vi "Marvin.vi"() -> ()   [LabVIEW 2017]
uses:
  Marvin ATP Remake 1.5.18/PCAN_Driver/ControlCAN.llb/CAN Channel.ctl
  Marvin ATP Remake 6.5.18 - Copy/PCAN_Driver/ControlCAN.llb/DevType.ctl
  Marvin ATP Remake 6.5.18/PCAN_Driver/ControlCAN.llb/VCI_INIT_CONFIG.ctl
  Marvin ATP Remake 6.5.18/PCAN_Driver/ControlCAN.llb/InitFlag.ctl
  Marvin ATP Remake 6.5.18/PCAN_Driver/ControlCAN.llb/Fliter.ctl
  Marvin ATP Remake 6.5.18/PCAN_Driver/ControlCAN.llb/Mode.ctl
  <vilib>/Utility/miscctls.llb/LVMinMaxIncTypeDef.ctl
  PCAN_Driver/ControlCAN.llb/VCI_CAN_OBJ.ctl
  PCAN_Driver/ControlCAN.lvlib
panel:
  in  "Clear Data Array":bool
  in  "PlayPause Data Array":bool
  out "CAN Data":cluster{"Frame Data":u64, "Frame ID":u32}[](array[cluster]) {"Frame ID" format="%.0x"; "Frame Data" format="%016x"}
  out "Waveform Chart":dbl[](graph)
  in  "Help Button":bool
  in  "Clear Monitor":bool
  out "Array":u64[][](array[numeric]) format="%016x"
  out "Ambient Over temp":bool
  out "Ambient Sensor temp":bool
  out "Ambient Temperature":dbl
  in  "Motor Over Temp":bool
  in  "Speed control":bool
  out "Unit Adress":string
  in  "Serial Send":bool
  in  "Index":u16(ring) items=["1"=1, "2"=2, "3"=3]
  out "read buffer":string
  in  "SetGet":enum16{"Get", "Set"}(ring)
  in  "Function":T1(ring)
  in  "Value":dbl
  in  "Value 1/2":enum16{"1", "2"}(ring)
  out "Msg Count":u32
  in  "Param to Set":u16(ring) items=["EBAY 5F"=95, "AHU 3F"=63, "AHU 2F"=47]
  out "UUT":u8
  out "Horizontal Progress Bar":i32(slide) min=0 max=48 scale=0.0..50.0
  in  "Set Param.":bool
  in  "Serial Monitor":bool caption="Graph Button"
  in  "Serial Com":bool
  in  "VISA resource name":refnum<visa-resource-name>="COM6"
  out "Serial Status":bool
  in  "Graph Button":bool
  in  "Refresh Button":bool
  out "Data Send":u64 format="%016x"
  in  "Motor Speed RPM":u16
  out "Under voltage/Over voltage":bool
  out "Speed error":bool
  out "Derated drive temp":bool
  out "Motor Over temperature":bool
  out "Commutation err":bool
  out "Motor Sensor temp Fauilre":bool
  out "Drive Over temperature":bool
  out "Drive Sensor temp Failure":bool
  out "Motor Phase Current RMS":dbl
  out "ECS State":u16
  out "Motor Speed RPM":dbl
  out "Motor Stator Temp.":dbl
  out "Power transistor Heat sink Temp.":dbl
  out "DC Current":dbl
  out "DC Voltage":dbl
  in  "Can Send":bool
  in  "Stop":bool
  out "Config_CANAT":T8 {"DevType" items=["USB-CAN"=3, "USB-CAN2"=4]; "CanIndex" items=["通道1", "通道2"]; "VCI_INIT_CONFIG"."Fliter" items=["接收所有类型"=3, "只接收标准帧"=4, "只接收扩展帧"=7]; "VCI_INIT_CONFIG"."Mode" items=["正常工作", "自测模式（环回）", "仅侦听模式"]; "VCI_INIT_CONFIG"."InitFlag" items=["使用Flash参数", "使用界面设置参数"]}
  in  "Channel 2":T3 caption="Channel" items=["Channel 1", "Channel 2"]
  out "CAN Status":bool
  out "Driver Version":string
  out "Hall Sensor Fault":bool
  out "Motor Phase Current":u16
  in  "Motor Phase Current":u16
  # "ver 1.7b"
  # "Marvin"
  # "REDLER TECHNOLOGIES LTD"
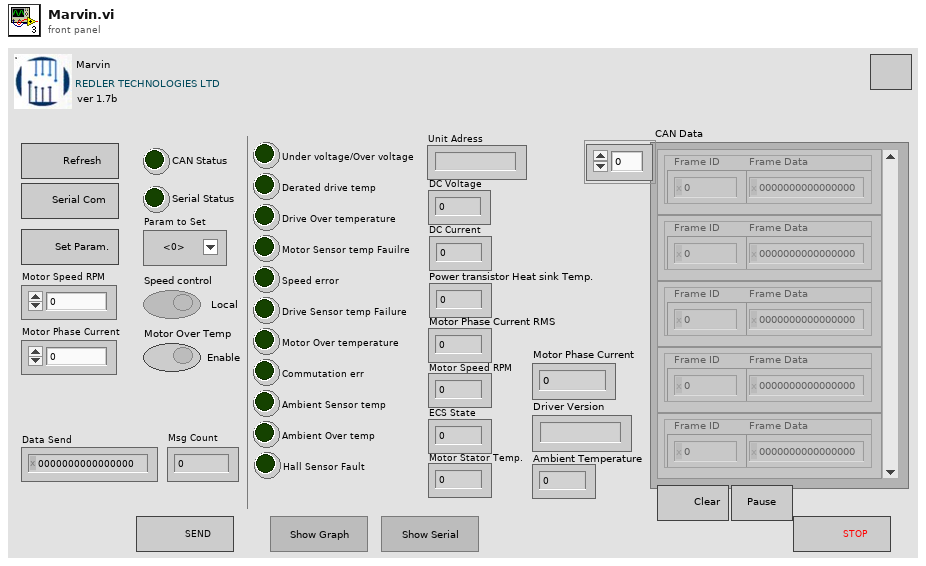
[diagram p1: front panel]
types:
  T1 = enum16{"Enable Conf. EP=1", "Serial Number", "Temperature", "Unit Adress", "Calibration", "Velocity", "Version"}
  T2 = typedef "ControlCAN.lvlib/DevType.ctl" = u32
  T3 = typedef "ControlCAN.lvlib/CAN Channel.ctl" = u32
  T4 = typedef "ControlCAN.lvlib/VCI_INIT_CONFIG.ctl" = cluster{"AccCode":u32, "AccMask":u32, "InitFlag":T5, "Fliter":T6, "Timing0":u8, "Timing1":u8, "Mode":T7}
  T5 = typedef "ControlCAN.lvlib/InitFlag.ctl" = u32
  T6 = typedef "ControlCAN.lvlib/Fliter.ctl" = u8
  T7 = typedef "ControlCAN.lvlib/Mode.ctl" = u8
  T8 = cluster{"DevType":T2, "DevIndex":u32, "CanIndex":T3, "VCI_INIT_CONFIG":T4}
  T9 = cluster{"ID":u32, "MSGTYPE":u8, "LEN":u8, "aDATA":u8[]}[]
  T10 = cluster{"ID":u32, "MSGTYPE":u8, "LEN":u8, "aDATA":u8[]}
  T11 = enum8{"Enabled", "Disabled", "Disabled and Grayed Out"}
  T12 = typedef "LVMinMaxIncTypeDef.ctl" = cluster{"Minimum":dbl, "Maximum":dbl, "Increment":dbl}
  T13 = enum32{"Invalid", "Standard", "Closed", "Hidden", "Minimized", "Maximized"}
  T14 = typedef "ControlCAN.lvlib/VCI_CAN_OBJ.ctl" = cluster{"ID":u32, "TimeStamp":u32, "TimeFlag":u8, "SendType":u8, "RemoteFlag":u8, "ExternFlag":u8, "DataLen":u8, "Data":u8[], "Reserved":u8[]}
  T15 = cluster{"Type":enum16{"接收", "发送"}, "Channel":T3, "Time":timestamp, "VCI_CAN_OBJ":T14}[]
  T16 = cluster{"Type":enum16{"接收", "发送"}, "Channel":T3, "Time":timestamp, "VCI_CAN_OBJ":T14}
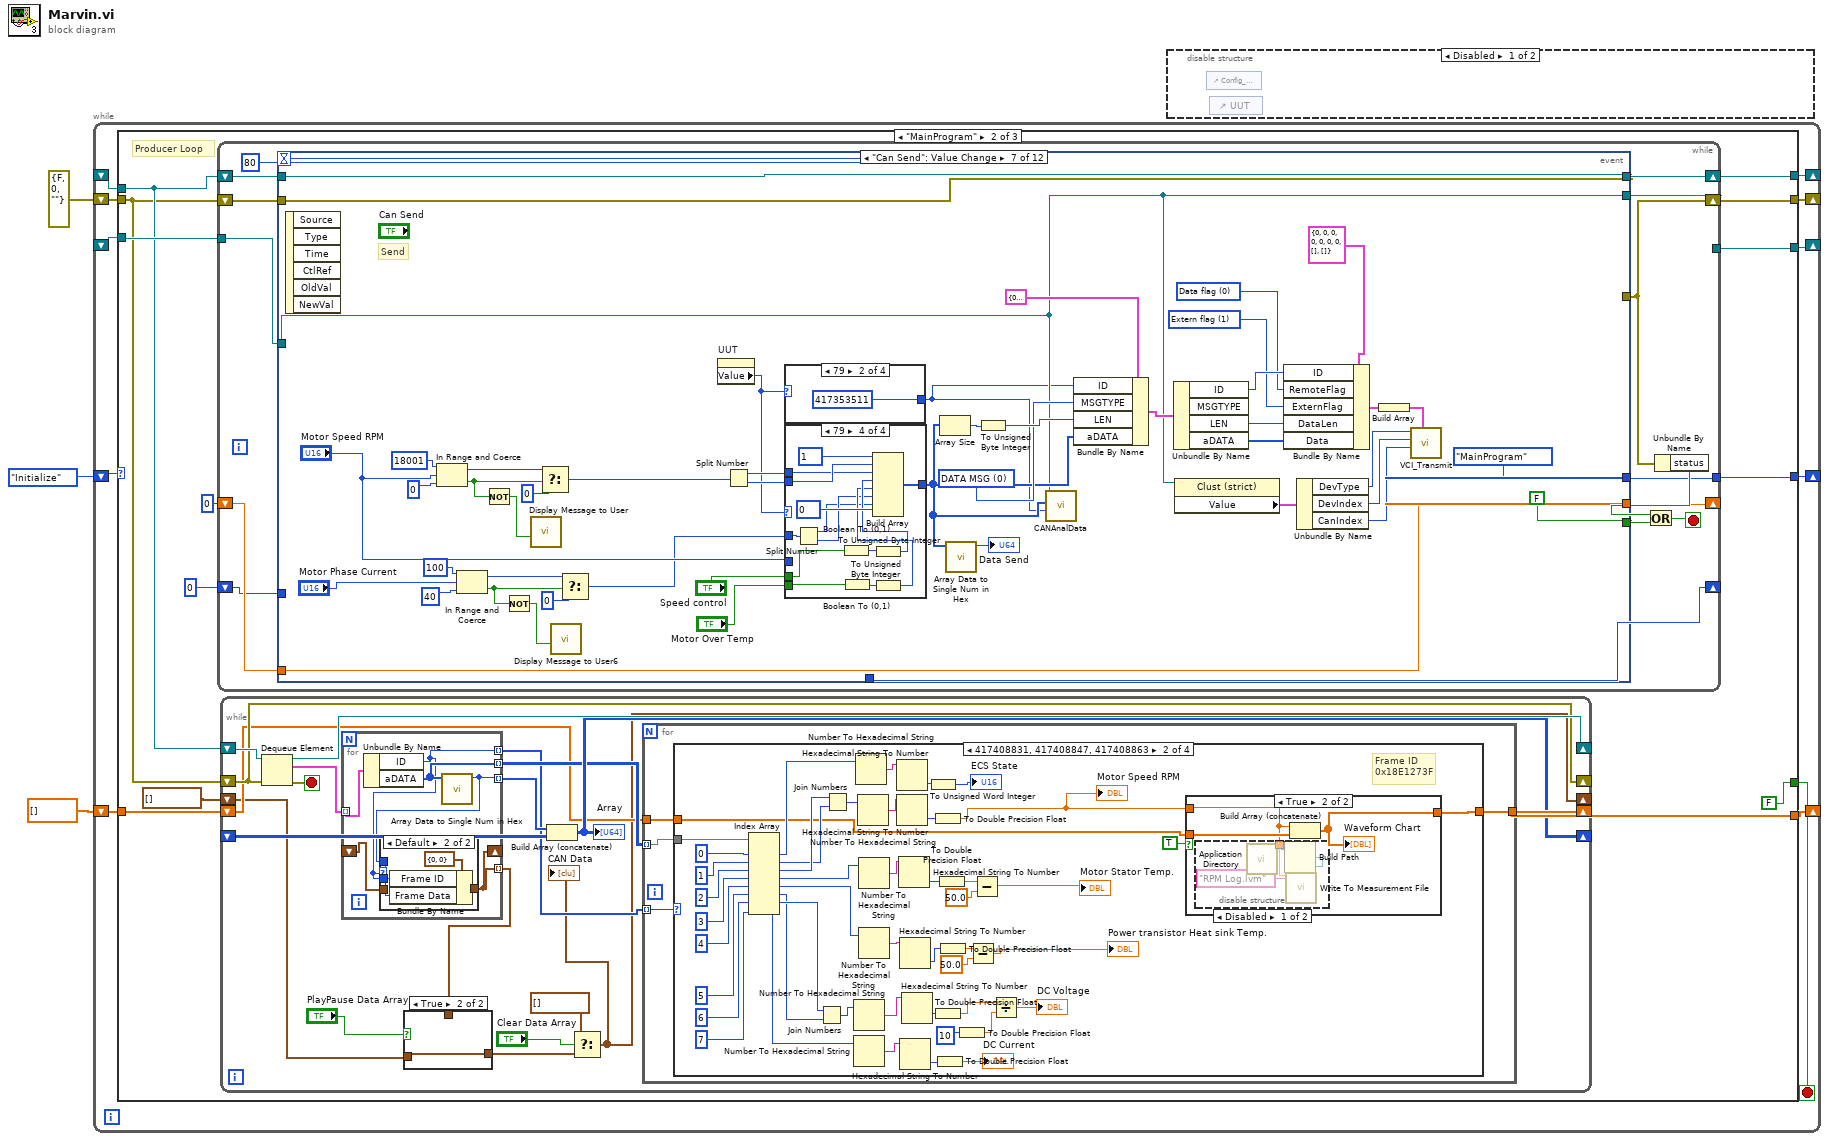
[diagram p0: block diagram]
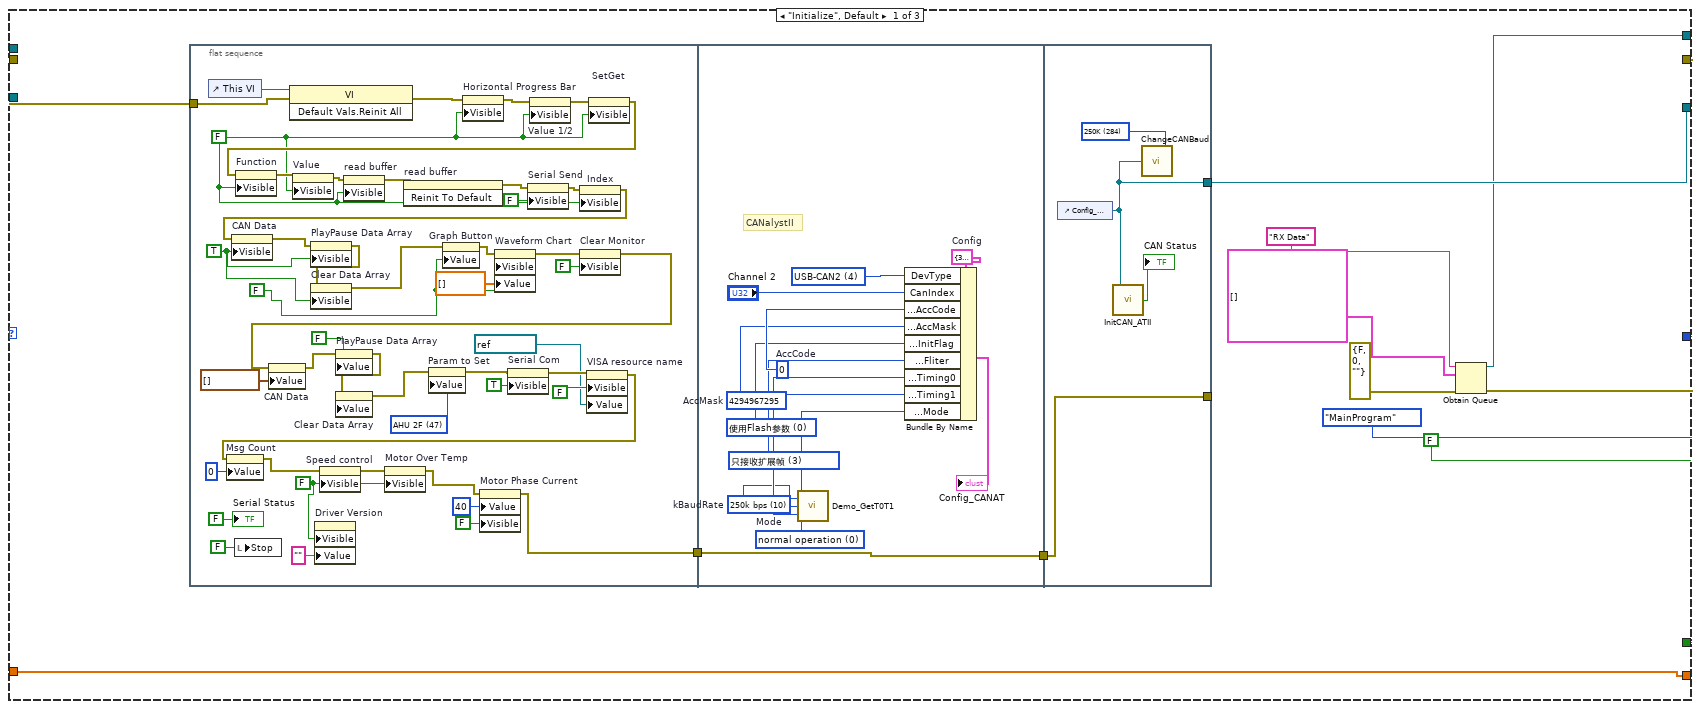
[diagram p3: hidden frame]
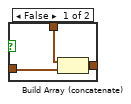
[diagram p4: hidden frame]
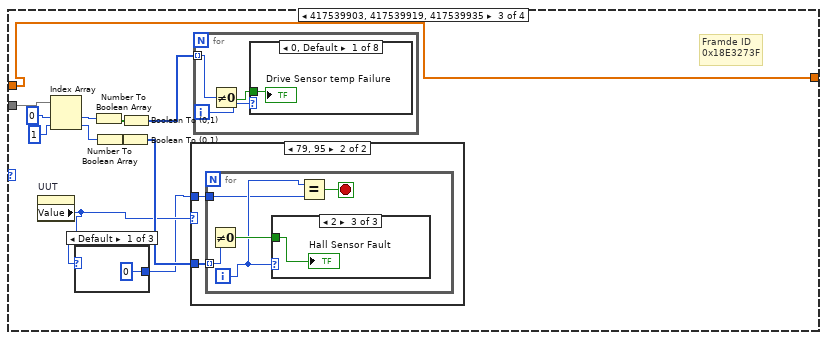
[diagram p8: hidden frame]
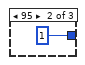
[diagram p9: hidden frame]
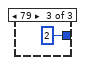
[diagram p10: hidden frame]
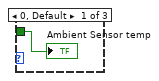
[diagram p12: hidden frame]
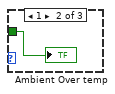
[diagram p13: hidden frame]
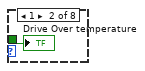
[diagram p14: hidden frame]
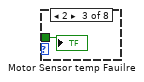
[diagram p15: hidden frame]
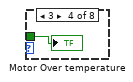
[diagram p16: hidden frame]
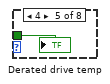
[diagram p17: hidden frame]
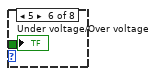
[diagram p18: hidden frame]
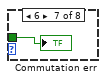
[diagram p19: hidden frame]
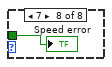
[diagram p20: hidden frame]
diagram:
  n1 = while {
    shift-right: [w9] -> _
    shift-left: enum16{"Stop", "MainProgram", "Initialize"}."Initialize" -> [w14]
    shift-right: [w13] -> _
    shift-left: _ -> [w12]
    shift-right: [w11] -> _
    shift-left: _ -> [w8]
    shift-right: [w10] -> _
    shift-left: errorcluster {"status"=FALSE, "code"=0, "source"=""} ("error out") -> [w7]
    shift-right: [w4] -> _
    shift-left: dbl[] [] -> [w5]
    stop <- w6 stop-if-true
    n2 = case shown="\"MainProgram\"" w14 {
      tunnel: [w26 w100 w995] -> w13
      tunnel: w12 -> [_ w103 w995]
      tunnel: [w22 w102 w996] -> w11
      tunnel: [w21 w101 w997] -> w10
      tunnel: [enum16{"Stop", "MainProgram", "Initialize"}."MainProgram" w99 enum16{"Stop", "MainProgram", "Initialize"}."Stop"] -> w9
      tunnel: w8 -> [_ w98 w996]
      tunnel: w7 -> [w19 w97 w998]
      tunnel: [FALSE ("Stop") FALSE ("Stop") w994] -> w6
      tunnel: w5 -> [w15 w94 w992]
      tunnel: [w15 w93 w992] -> w4
      frame "Initialize", Default {
        n3 = flat-sequence {
          tunnel: w19 -> [w55]
          tunnel: [w29] -> w17
          tunnel: [w74] -> w18
          tunnel: w17 -> [w74]
          tunnel: [w88] -> w26
          tunnel: w18 -> [w87]
          tunnel: [w87] -> _
          frame #0 {
            w38 = FALSE ("PlayPause Data Array")
            w32 = FALSE ("Visible")
            w65 = u16 47 items=["EBAY 5F"=95, "AHU 3F"=63, "AHU 2F"=47] ("Param to Set")
            w33 = TRUE ("Visible")
            w49 = FALSE ("Visible")
            w37 = FALSE ("Graph Button")
            n4 = control-ref of="This VI"() -> (w73:refnum<vi>)
            n5 = local write "Stop"(FALSE ("Stop")) -> ()
            n6 = invoke class="VI" method="Default Vals.Reinit All"(reference=w73, error in=w55) -> (error out=w54:errorcluster)  [unwired: 1 in, 2 out]
            n7 = property on="Driver Version" class="Str"("Visible"=w32, "Value"="" ("Driver Version")) -> ()  [unwired: 2 in, 2 out]
            n8 = property on="Horizontal Progress Bar" class="Slide (strict)"(error in=w54, "Visible"=w49) -> (error out=w63:errorcluster)  [unwired: 1 in, 1 out]
            n9 = property on="Value 1/2" class="Enum (strict)"(error in=w63, "Visible"=w49) -> (error out=w62:errorcluster)  [unwired: 1 in, 1 out]
            n10 = property on="SetGet" class="Enum (strict)"(error in=w62, "Visible"=w49) -> (error out=w61:errorcluster)  [unwired: 1 in, 1 out]
            n11 = property on="Function" class="Enum (strict)"(error in=w61, "Visible"=w49) -> (error out=w60:errorcluster)  [unwired: 1 in, 1 out]
            n12 = property on="Value" class="DigNum (strict)"(error in=w60, "Visible"=w49) -> (error out=w59:errorcluster)  [unwired: 1 in, 1 out]
            n13 = property on="read buffer" class="Str"(error in=w59, "Visible"=w49) -> (error out=w51:errorcluster)  [unwired: 1 in, 1 out]
            n14 = invoke on="read buffer" class="Str" method="Reinit To Default"(error in=w51) -> (error out=w50:errorcluster)  [unwired: 2 in, 2 out]
            n15 = property on="Serial Send" class="Bool (strict)"(error in=w50, "Visible"=FALSE) -> (error out=w58:errorcluster)  [unwired: 1 in, 1 out]
            n16 = property on="Index" class="Ring (strict)"(error in=w58, "Visible"=w49) -> (error out=w44:errorcluster)  [unwired: 1 in, 1 out]
            n17 = property on="CAN Data" class="Arr (strict)"(error in=w44, "Visible"=w33) -> (error out=w36:errorcluster)  [unwired: 1 in, 1 out]
            n18 = property on="PlayPause Data Array" class="Bool (strict)"(error in=w36, "Visible"=w33) -> (error out=w35:errorcluster)  [unwired: 1 in, 1 out]
            n19 = property on="Clear Data Array" class="Bool (strict)"(error in=w35, "Visible"=w33) -> (error out=w34:errorcluster)  [unwired: 1 in, 1 out]
            n20 = property on="Graph Button" class="Bool (strict)"(error in=w34, "Value"=w37) -> (error out=w47:errorcluster)  [unwired: 1 in, 1 out]
            n21 = property on="Waveform Chart" class="WFChart (strict)"(error in=w47, "Visible"=w37, "Value"=dbl[] [] ("Waveform Chart")) -> (error out=w46:errorcluster)  [unwired: 1 in, 1 out]
            n22 = property on="Clear Monitor" class="Bool"(error in=w46, "Visible"=FALSE) -> (error out=w43:errorcluster)  [unwired: 1 in, 1 out]
            n23 = property on="CAN Data" class="Arr (strict)"(error in=w43, "Value"=cluster{"Frame Data":u64, "Frame ID":u32}[] [] ("CAN Data")) -> (error out=w41:errorcluster)  [unwired: 1 in, 1 out]
            n24 = property on="PlayPause Data Array" class="Bool (strict)"(error in=w41, "Value"=w38) -> (error out=w40:errorcluster)  [unwired: 1 in, 1 out]
            n25 = property on="Clear Data Array" class="Bool (strict)"(error in=w40, "Value"=w38) -> (error out=w39:errorcluster)  [unwired: 1 in, 1 out]
            n26 = property on="Param to Set" class="Ring (strict)"(error in=w39, "Value"=w65) -> (error out=w57:errorcluster)  [unwired: 1 in, 1 out]
            n27 = property on="Serial Com" class="Bool"(error in=w57, "Visible"=TRUE) -> (error out=w70:errorcluster)  [unwired: 1 in, 1 out]
            n28 = property on="VISA resource name" class="VISAName"(error in=w70, "Visible"=FALSE, "Value"=refnum<visa-resource-name> "COM1" ("VISA resource name")) -> (error out=w56:errorcluster)  [unwired: 1 in, 1 out]
            n29 = property on="Msg Count" class="DigNum (strict)"(error in=w56, "Value"=u32 0 ("Msg Count")) -> (error out=w53:errorcluster)  [unwired: 1 in, 1 out]
            n30 = property on="Speed control" class="Bool (strict)"(error in=w53, "Visible"=w32) -> (error out=w52:errorcluster)  [unwired: 1 in, 1 out]
            n31 = property on="Motor Over Temp" class="Bool (strict)"(error in=w52, "Visible"=w32) -> (error out=w30:errorcluster)  [unwired: 1 in, 1 out]
            n32 = property on="Motor Phase Current" class="DigNum (strict)"(error in=w30, "Value"=u16 40 ("Motor Phase Current"), "Visible"=FALSE) -> (error out=w29:errorcluster)  [unwired: 1 in, 1 out]
            "Serial Status" <- FALSE ("Serial Status")
          }
          frame #1 {
            w78 = u32 4294967295  # AccMask
            w77 = T5 0 items=["使用Flash参数", "使用界面设置参数"] ("InitFlag")
            w75 = T7 0 items=["normal operation", "Listen-only mode", "test mode"]  # Mode
            w76 = T6 3 items=["接收所有类型"=1, "只接收标准帧"=2, "只接收扩展帧"=3] ("Fliter")
            w82 = u8 10 items=["5k bps"=1, "10k bps"=2, "20k bps"=3, "40k bps"=4, "50k bps"=5, "80k bps"=6, "100k bps"=7, "125k bps"=8, "200k bps"=9, "250k bps"=10, "400k bps"=11, "500k bps"=12, "666k bps"=13, "800k bps"=14, "1000k bps"=15, "33.33k bps"=16, "66.66k bps"=17, "83.33k bps"=18]  # kBaudRate
            w79 = u32 0  # AccCode
            w80 = T2 4 items=["USB-CAN"=3, "USB-CAN2"=4] ("DevType")
            w81 = T8 {"DevType"=3, "DevIndex"=0, "CanIndex"=0, "VCI_INIT_CONFIG"={"AccCode"=0, "AccMask"=0, "InitFlag"=1, "Fliter"=7, "Timing0"=0, "Timing1"=0, "Mode"=0}}  # Config
            # "CANalystII"
            n33 = call "Demo_GetT0T1.vi"("kBaudRate"=w82) -> ("Timing0"=w84:u8, "Timing1"=w85:u8)
            n34 = Bundle By Name(cluster=w81, "DevType"=w80, "CanIndex"="Channel 2", "VCI_INIT_CONFIG.AccCode"=w79, "VCI_INIT_CONFIG.AccMask"=w78, "VCI_INIT_CONFIG.InitFlag"=w77, "VCI_INIT_CONFIG.Fliter"=w76, "VCI_INIT_CONFIG.Timing0"=w84, "VCI_INIT_CONFIG.Timing1"=w85, "VCI_INIT_CONFIG.Mode"=w75) -> (→"Config_CANAT":T8)
          }
          frame #2 {
            w89 = u16 284 items=["1M"=20, "500K"=28, "250K"=284, "125K"=796, "100K"=17199, "50K"=18223, "20K"=21295, "10K"=26415, "5K"=32639] ("baud in")
            n35 = control-ref of="Config_CANAT"() -> (w88:refnum<vi>)
            n36 = call "InitCAN_ATII.vi"("Config"=w88) -> ("Sts"=→"CAN Status":bool)
            n37 = call "ChangeCANBaud.vi"("baud in"=w89, "reference"=w88) -> ()
          }
        }
        n38 = Obtain Queue(name (unnamed)="RX Data", element data type=T9 [], error in (no error)=errorcluster {"status"=FALSE, "code"=0, "source"=""}) -> (queue out=w22:refnum<queue>, error out=w21:errorcluster)  [unwired: 2 in, 1 out]
      }
      frame "MainProgram" {
        # "Producer Loop"
        n39 = while {
          shift-right: [w268] -> w101
          shift-left: w97 -> [w270]
          shift-right: [w269] -> w102
          shift-left: w98 -> [w271]
          tunnel: w103 -> [w272]
          tunnel: [w265] -> w100
          tunnel: [w264] -> w99
          shift-right: [w262] -> _
          shift-left: 0 -> [w263]
          shift-right: [w260] -> _
          shift-left: 0 -> [w261]
          stop <- w273 stop-if-true
          n40 = event shown="[6] \"Can Send\": Value Change" {
            selector: _ -> [_ _ _ _ _ _ _ _ _ _ _ _]
            dyn-events: _ -> [_ _ _ _ _ _ _ _ _ _ _ _]
            timeout: 80 ("Numeric") -> [_ _ _ _ _ _ _ _ _ _ _ _]
            tunnel: w272 -> [w294 w372 w391 w458 w713 w811 w841 w932 w952 w969 w984 w990]
            tunnel: w271 -> [w291 w373 w394 w459 w712 w812 w862 w933 w951 w970 w981 w987]
            tunnel: w270 -> [w276 w371 w389 w446 w705 w804 w861 w912 w947 w962 w980 w988]
            tunnel: [w289 w373 w394 w459 w712 w812 w862 w933 w951 w970 w979 w987] -> w269
            tunnel: [w288 w366 w390 w451 w701 w801 w861 w919 w944 w960 w977 w986] -> w268
            tunnel: [FALSE ("Stop") FALSE ("Stop") FALSE ("Stop") FALSE ("Stop") FALSE ("Stop") FALSE ("Stop") FALSE ("Stop") FALSE ("Stop") FALSE ("Stop") FALSE ("Stop") TRUE ("Stop") TRUE ("Stop")] -> w266
            tunnel: [w287 w372 w391 w458 w713 w811 w841 w932 w952 w969 w984 w990] -> w265
            tunnel: [enum16{"Stop", "MainProgram", "Initialize"}."MainProgram" enum16{"Stop", "MainProgram", "Initialize"}."MainProgram" enum16{"Stop", "MainProgram", "Initialize"}."MainProgram" enum16{"Stop", "MainProgram", "Initialize"}."MainProgram" enum16{"Stop", "MainProgram", "Initialize"}."MainProgram" enum16{"Stop", "MainProgram", "Initialize"}."MainProgram" enum16{"Stop", "MainProgram", "Initialize"}."MainProgram" enum16{"Stop", "MainProgram", "Initialize"}."MainProgram" enum16{"Stop", "MainProgram", "Initialize"}."MainProgram" enum16{"Stop", "MainProgram", "Initialize"}."MainProgram" enum16{"Stop", "MainProgram", "Initialize"}."Stop" enum16{"Stop", "MainProgram", "Initialize"}."Initialize"] -> w264
            tunnel: w263 -> [w283 w376 w387 w447 w703 w815 w827 w928 w943 w958 w976 w985]
            tunnel: [w282 w376 w387 w447 w703 w815 w827 w928 w943 w958 w976 w985] -> w262
            tunnel: w261 -> [w275 _ _ _ _ _ _ _ _ _ _ _]
            tunnel: [w275 _ _ _ _ _ _ _ _ _ _ _] -> w260
            event Timeout {
              n41 = event-data() -> ()  [unwired: 1 in, 3 out]
              n42 = property class="Clust (strict)"(reference=w294) -> (reference out=w287:refnum<vi>, "Value"=w295:T8)  [unwired: 1 in, 1 out]
              n43 = property on="Speed control" class="Bool (strict)"(error in=w276) -> ("Value"=w277:bool)  [unwired: 1 in, 2 out]
              n44 = case shown="True" w277 {
                frame False {
                }
                frame True {
                  n45 = property on="Motor Speed RPM" class="DigNum (strict)"() -> ("Value"=w301:u16)  [unwired: 2 in, 2 out]
                  n46 = control-ref of="Config_CANAT"() -> (w300:refnum<vi>)
                  n47 = control-ref of="UUT"() -> (w299:refnum<vi>)
                  n48 = call "CANSendMotorSpeed.vi"("Remote"=TRUE, "Motor Speed RPM"=w301, "UUT"=w299, "CAN Cluster in"=w300) -> ()  [unwired: 7 in, 1 out]
                }
              }
              n49 = Unbundle By Name(w295) -> ("DevType"=w296:T2, "CanIndex"=w292:T3)
              n50 = property on="Horizontal Progress Bar" class="Slide (strict)"(error in=w276, "Visible"=FALSE) -> (error out=w278:errorcluster)  [unwired: 1 in, 1 out]
              n51 = call "VCI_Receive.vi"("CANIndex"=w292, "DevIndex"=u32 0, "DevType"=w296) -> ("Recieve"=w290:T14[])  [unwired: 3 in, 5 out]
              n52 = Empty Array?(array=w290) -> (empty?=w293:bool)
              n53 = case shown="False" w293 {
                tunnel: w292 -> [w313 _]
                tunnel: w287 -> [w311 _]
                tunnel: w291 -> [w310 w365]
                tunnel: w278 -> [w309 w364]
                tunnel: w290 -> [w314 _]
                tunnel: [w304 w364] -> w288
                tunnel: [w303 w365] -> w289
                tunnel: [w302 0] -> w279
                frame False {
                  n54 = call "Demo_MakeDispBuff.vi"("Channel"=w313, "Type"=enum16{"接收", "发送"}."接收", "OBJs"=w314) -> ("Buffer"=w312:T15)
                  n55 = for {
                    N: 3 -> [_]
                    tunnel: w312 -> [w328]
                    tunnel: w311 -> [w327]
                    tunnel: w310 -> [w318]
                    tunnel: w309 -> [w317]
                    tunnel: [w320] -> w307 mode=indexing
                    tunnel: [w318] -> w306
                    tunnel: [w317] -> w305
                    tunnel: [w316] -> w302
                    i -> [w316]
                    n56 = property class="Clust (strict)"(reference=w327) -> ("Value"=w325:T8)  [unwired: 1 in, 2 out]
                    n57 = Index Array(array=w328, index=w316) -> (element=w321:T16)
                    n58 = Unbundle By Name(w321) -> ("Channel"=w323:T3, "VCI_CAN_OBJ"=w326:T14)  [unwired: 2 out]
                    n59 = Unbundle By Name(w325) -> ("CanIndex"=w324:T3)
                    n60 = Equal?(x=w324, y=w323) -> (x = y?=w322:bool)
                    n61 = case shown="True" w322 {
                      tunnel: w326 -> [_ w344]
                      tunnel: [w329 w340] -> w320
                      tunnel: T10 {"ID"=0, "MSGTYPE"=0, "LEN"=0, "aDATA"=[]} ("Msg") -> [w329 w339]
                      frame False {
                      }
                      frame True {
                        n62 = Unbundle By Name(w344) -> ("ID"=w338:u32, "DataLen"=w343:u8, "Data"=w341:u8[])
                        n63 = Bundle By Name(cluster=w339, "ID"=w338, "MSGTYPE"=u8 0, "LEN"=w343, "aDATA"=w341) -> (w340:T10)
                        n64 = Unbundle By Name(w340) -> ("ID"=w336:u32)
                        n65 = Split Number(x=w336) -> (lo(x)=w337:u16)  [unwired: 1 out]
                        n66 = Split Number(x=w337) -> (lo(x)=w334:u8)  [unwired: 1 out]
                        "UUT" <- w334
                        n67 = case shown="95" w334 {
                          tunnel: ["EBAY 5F" "PUMP 4F" w357 "AHU 3F" "AHU 2F"] -> w333
                          tunnel: [TRUE w354 w358 w359 w361] -> w331
                          tunnel: [TRUE w354 w356 w359 w361] -> w330
                          frame 95 {
                          }
                          frame 79 {
                            w354 = TRUE
                          }
                          frame Default {
                            n68 = property on="Hall Sensor Fault" class="Bool (strict)"() -> ("Visible"=w356:bool)  [unwired: 2 in, 2 out]
                            n69 = property on="Speed control" class="Bool (strict)"() -> ("Visible"=w358:bool)  [unwired: 2 in, 2 out]
                            n70 = property on="Unit Adress" class="Str"() -> ("Value"=w357:string)  [unwired: 2 in, 2 out]
                          }
                          frame 63 {
                            w359 = FALSE
                          }
                          frame 47 {
                            w361 = FALSE
                          }
                        }
                        n71 = Not Equal To 0?(x=w334) -> (x != 0?=w335:bool)
                        n72 = case shown="True" w335 {
                          tunnel: w334 -> [_ w350]
                          tunnel: w333 -> [_ w347]
                          tunnel: [w345 w346] -> w332
                          frame False {
                            n73 = property on="Unit Adress" class="Str"() -> ("Value"=w345:string)  [unwired: 2 in, 2 out]
                          }
                          frame True {
                            n74 = Number To Decimal String(number=w350) -> (decimal integer string=w349:string)  [unwired: 1 in]
                            n75 = call <vilib>:"Space Constant.vi"() -> ("String"=w348:string)
                            n76 = Concatenate Strings(w349, w348, w347) -> (w346:string)
                          }
                        }
                        "Unit Adress" <- w332
                        n77 = property on="Driver Version" class="Str"("Visible"=w331) -> ()  [unwired: 2 in, 2 out]
                        n78 = property on="Hall Sensor Fault" class="Bool (strict)"("Visible"=w330) -> ()  [unwired: 2 in, 2 out]
                        n79 = property on="Motor Phase Current" class="DigNum (strict)"("Visible"=w330) -> ()  [unwired: 2 in, 2 out]
                        n80 = property on="Motor Phase Current" class="DigNum (strict)"("Visible"=w330) -> ()  [unwired: 2 in, 2 out]
                        n81 = property on="Ambient Over temp" class="Bool (strict)"("Visible"=w331) -> ()  [unwired: 2 in, 2 out]
                        n82 = property on="Ambient Sensor temp" class="Bool (strict)"("Visible"=w331) -> ()  [unwired: 2 in, 2 out]
                        n83 = property on="Ambient Temperature" class="DigNum (strict)"("Visible"=w331) -> ()  [unwired: 2 in, 2 out]
                        n84 = property on="Motor Over Temp" class="Bool (strict)"("Visible"=w331) -> ()  [unwired: 2 in, 2 out]
                        n85 = property on="Speed control" class="Bool (strict)"("Visible"=w331) -> ()  [unwired: 2 in, 2 out]
                      }
                    }
                  }
                  n86 = Enqueue Element(queue=w306, element=w307, error in (no error)=w305) -> (queue out=w303:refnum<queue>, error out=w304:errorcluster)  [unwired: 2 out]
                }
                frame True {
                }
              }
              n87 = Divide(x=w279, y=u32 2) -> (x/y=w280:dbl)
              n88 = Add(x=w280, y=w283) -> (x+y=w282:dbl)
              "Msg Count" <- w282
            }
            event "Clear Monitor": Value Change {
              n89 = event-data() -> ()  [unwired: 1 in, 6 out]
              n90 = property on="VISA resource name" class="VISAName"(error in=w371) -> (error out=w370:errorcluster, "Value"=w369:refnum<visa-resource-name>)  [unwired: 1 in, 1 out]
              n91 = disable-structure shown="Enabled" {
                disable-tunnel: w370 -> [w381 w384]
                disable-tunnel: w369 -> [w379 w385]
                disable-tunnel: [w378 ""] -> w368
                disable-tunnel: [w377 w383] -> w367
                frame Disabled {
                  n92 = call "Serial.vi"("error in (no error)"=w381, "Clear Log"=TRUE, "VISA resource name"=w379) -> ("error out"=w377:errorcluster, "read buffer"=w378:string)  [unwired: 7 in]
                }
                frame Enabled {
                  n93 = VISA Flush I/O Buffer(VISA resource name=w385, error in (no error)=w384) -> (error out=w383:errorcluster)  [unwired: 1 in, 1 out]
                }
              }
              n94 = property on="read buffer" class="Str"(error in=w367, "Value"=w368) -> (error out=w366:errorcluster)  [unwired: 1 in, 1 out]
            }
            event "Serial Monitor": Value Change {
              n95 = event-data() -> ()  [unwired: 1 in, 6 out]
              n96 = property on="Serial Status" class="Bool (strict)"(error in=w389) -> (error out=w388:errorcluster, "Value"=w386:bool)  [unwired: 1 in, 1 out]
              n97 = case shown="True" w386 {
                tunnel: w388 -> [w398 w411]
                tunnel: [w396 w416] -> w390
                frame False {
                  n98 = call "Display Message to User3"("error in (no error)"=w398) -> ("error out"=w397:errorcluster)  [unwired: 9 in, 1 out]
                  n99 = property on="Serial Monitor" class="Bool (strict)"(error in=w397, "Value"=FALSE ("Serial Monitor")) -> (error out=w396:errorcluster)  [unwired: 1 in, 1 out]
                }
                frame True {
                  w403 = FALSE ("Visible")
                  w413 = FALSE ("Visible")
                  w414 = u16 1 items=["1"=1, "2"=2, "3"=3] ("Index")
                  n100 = property on="Index" class="Ring (strict)"(error in=w411, "Value"=w414) -> (error out=w410:errorcluster)  [unwired: 1 in, 1 out]
                  n101 = property on="Value 1/2" class="Enum (strict)"(error in=w410, "Visible"=w413) -> (error out=w409:errorcluster)  [unwired: 1 in, 1 out]
                  n102 = property on="Value" class="DigNum (strict)"(error in=w409, "Visible"=w413) -> (error out=w408:errorcluster)  [unwired: 1 in, 1 out]
                  n103 = property on="SetGet" class="Enum (strict)"(error in=w408, "Value"=enum16{"Get", "Set"}."Get" ("SetGet")) -> (error out=w407:errorcluster)  [unwired: 1 in, 1 out]
                  n104 = property on="Serial Send" class="Bool (strict)"(error in=w407, "Visible"=w403) -> (error out=w402:errorcluster)  [unwired: 1 in, 1 out]
                  n105 = property on="Clear Monitor" class="Bool"(error in=w402, "Visible"=w403) -> (error out=w401:errorcluster)  [unwired: 1 in, 1 out]
                  n106 = property on="Function" class="Enum (strict)"(error in=w401, "Value"=T1."Serial Number" ("Function")) -> (error out=w406:errorcluster)  [unwired: 1 in, 1 out]
                  n107 = property on="Index" class="Ring (strict)"(error in=w406, "DisabledEnum"=T11."Disabled and Grayed Out" ("Disabled")) -> (error out=w404:errorcluster)  [unwired: 1 in, 1 out]
                  n108 = case shown="True" "Serial Monitor" {
                    selector: "Serial Monitor" -> [w420 w441]
                    tunnel: w404 -> [w419 w437]
                    tunnel: [w422 w438] -> w416
                    tunnel: [FALSE TRUE] -> w400
                    frame False {
                      n109 = property on="Graph Button" class="Bool (strict)"(error in=w419) -> (error out=w418:errorcluster, "Value"=w417:bool)  [unwired: 1 in, 1 out]
                      n110 = case shown="True" w417 {
                        tunnel: [w426 w431] -> w423
                        tunnel: w418 -> [w428 w434]
                        tunnel: w420 -> [w429 _]
                        frame False {
                          n111 = property on="Waveform Chart" class="WFChart (strict)"(error in=w428, "Visible"=FALSE) -> (error out=w425:errorcluster)  [unwired: 1 in, 1 out]
                          n112 = Not(x=w429) -> (.not. x?=w424:bool)
                          n113 = property on="PlayPause Data Array" class="Bool (strict)"("Visible"=w424) -> ()  [unwired: 2 in, 2 out]
                          n114 = property on="Clear Data Array" class="Bool (strict)"("Visible"=w424) -> ()  [unwired: 2 in, 2 out]
                          n115 = property on="CAN Data" class="Arr (strict)"(error in=w425, "Visible"=w424) -> (error out=w426:errorcluster)  [unwired: 1 in, 1 out]
                        }
                        frame True {
                          w430 = FALSE ("Visible")
                          n116 = property on="Waveform Chart" class="WFChart (strict)"(error in=w434, "Visible"=TRUE) -> (error out=w432:errorcluster)  [unwired: 1 in, 1 out]
                          n117 = property on="PlayPause Data Array" class="Bool (strict)"("Visible"=w430) -> ()  [unwired: 2 in, 2 out]
                          n118 = property on="Clear Data Array" class="Bool (strict)"("Visible"=w430) -> ()  [unwired: 2 in, 2 out]
                          n119 = property on="CAN Data" class="Arr (strict)"(error in=w432, "Visible"=w430) -> (error out=w431:errorcluster)  [unwired: 1 in, 1 out]
                        }
                      }
                      n120 = property on="Serial Monitor" class="Bool (strict)"(error in=w423, "Value"=w420) -> (error out=w422:errorcluster)  [unwired: 1 in, 1 out]
                    }
                    frame True {
                      n121 = Not(x=w441) -> (.not. x?=w435:bool)
                      n122 = property on="PlayPause Data Array" class="Bool (strict)"("Visible"=w435) -> ()  [unwired: 2 in, 2 out]
                      n123 = property on="CAN Data" class="Arr (strict)"(error in=w437, "Visible"=w435) -> (error out=w436:errorcluster)  [unwired: 1 in, 1 out]
                      n124 = property on="Clear Data Array" class="Bool (strict)"("Visible"=w435) -> ()  [unwired: 2 in, 2 out]
                      n125 = property on="Serial Monitor" class="Bool (strict)"(error in=w436, "Value"=w441) -> (error out=w440:errorcluster)  [unwired: 1 in, 1 out]
                      n126 = property on="Graph Button" class="Bool (strict)"(error in=w440, "Value"=w435) -> (error out=w439:errorcluster)  [unwired: 1 in, 1 out]
                      n127 = property on="Waveform Chart" class="WFChart (strict)"(error in=w439, "Visible"=w435) -> (error out=w438:errorcluster)  [unwired: 1 in, 1 out]
                    }
                  }
                  n128 = property on="SetGet" class="Enum (strict)"("Visible"=w400) -> ()  [unwired: 2 in, 2 out]
                  n129 = property on="Index" class="Ring (strict)"("Visible"=w400) -> ()  [unwired: 2 in, 2 out]
                  n130 = property on="Function" class="Enum (strict)"("Visible"=w400) -> ()  [unwired: 2 in, 2 out]
                  n131 = property on="Clear Monitor" class="Bool"("Visible"=w400) -> ()  [unwired: 2 in, 2 out]
                  n132 = property on="Serial Send" class="Bool (strict)"("Visible"=w400) -> ()  [unwired: 2 in, 2 out]
                  n133 = property on="read buffer" class="Str"("Visible"=w400) -> ()  [unwired: 2 in, 2 out]
                }
              }
            }
            event "Serial Send", "Function", "SetGet": Value Change {
              n134 = event-data() -> ()  [unwired: 1 in, 6 out]
              n135 = case shown="\"Enable Conf. EP=1\"" "Function" {
                tunnel: w446 -> [w465 w470 w477 w479 w482 w486 w488 w489]
                tunnel: [w464 w472 w476 w481 w484 w485 w488 w489] -> w444
                frame "Serial Number" {
                  n136 = property on="Index" class="Ring (strict)"(error in=w465, "DisabledEnum"=T11."Disabled and Grayed Out" ("Disabled")) -> (error out=w464:errorcluster)  [unwired: 1 in, 1 out]
                }
                frame "Temperature" {
                  n137 = property on="UUT" class="DigNum (strict)"() -> ("Value"=w467:u8)  [unwired: 2 in, 2 out]
                  n138 = case shown="95" w467 {
                    tunnel: [i32[] [2] ("Disabled Items []") i32[] [3] ("Disabled Items []")] -> w468
                    frame 47, 63, Default {
                    }
                    frame 95 {
                    }
                  }
                  n139 = property on="Index" class="Ring (strict)"(error in=w470, "DisabledEnum"=T11."Enabled" ("Disabled"), "Visible"=TRUE, "Disabled Items []"=w468) -> (error out=w472:errorcluster)  [unwired: 1 in, 1 out]
                }
                frame "Unit Adress" {
                  n140 = property on="Index" class="Ring (strict)"(error in=w477, "DisabledEnum"=T11."Enabled" ("Disabled"), "Visible"=TRUE) -> (error out=w476:errorcluster)  [unwired: 1 in, 1 out]
                }
                frame "Calibration" {
                  n141 = property on="Index" class="Ring (strict)"(error in=w479, "DisabledEnum"=T11."Disabled and Grayed Out" ("Disabled")) -> (error out=w481:errorcluster)  [unwired: 1 in, 1 out]
                }
                frame "Velocity" {
                  n142 = property on="Index" class="Ring (strict)"(error in=w482, "DisabledEnum"=T11."Disabled and Grayed Out" ("Disabled")) -> (error out=w484:errorcluster)  [unwired: 1 in, 1 out]
                }
                frame "Version" {
                  n143 = property on="Index" class="Ring (strict)"(error in=w486, "DisabledEnum"=T11."Disabled and Grayed Out" ("Disabled")) -> (error out=w485:errorcluster)  [unwired: 1 in, 1 out]
                }
                frame "Enable Conf. EP=1" {
                }
                frame Default {
                }
              }
              n144 = property on="VISA resource name" class="VISAName"() -> ("Value"=w460:refnum<visa-resource-name>)  [unwired: 2 in, 2 out]
              n145 = property on="read buffer" class="Str"(error in=w444) -> (error out=w453:errorcluster, "Text.Scroll Position"=w450:u32)  [unwired: 1 in, 1 out]
              n146 = case shown="\"Set\"" "SetGet" {
                tunnel: "Function" -> [w493 w592]
                tunnel: w460 -> [w499 w602]
                tunnel: w453 -> [w496 w591]
                tunnel: "Value" -> [_ w601]
                tunnel: "Value 1/2" -> [_ w599]
                tunnel: "Index" -> [w494 w596]
                tunnel: [w498 w594] -> w452
                tunnel: [w491 w593] -> w457
                tunnel: "Serial Send" -> [w490 w583]
                frame "Get", Default {
                  w497 = FALSE ("Visible")
                  n147 = property on="Value" class="DigNum (strict)"(error in=w496, "Visible"=w497) -> (error out=w495:errorcluster)  [unwired: 1 in, 1 out]
                  n148 = property on="Value 1/2" class="Enum (strict)"(error in=w495, "Visible"=w497) -> (error out=w492:errorcluster)  [unwired: 1 in, 1 out]
                  n149 = case shown="True" w490 {
                    tunnel: w499 -> [_ w510]
                    tunnel: [w500 w505] -> w498
                    tunnel: w494 -> [_ w509]
                    tunnel: w493 -> [_ w508]
                    tunnel: w492 -> [w500 w507]
                    tunnel: [w501 w503] -> w491
                    frame False {
                      n150 = property on="read buffer" class="Str"() -> ("Value"=w501:string)  [unwired: 2 in, 2 out]
                    }
                    frame True {
                      n151 = case shown="\"Serial Number\"" w508 {
                        tunnel: w510 -> [w515 w533 w549 w558 w565 w576 _]
                        tunnel: w507 -> [w513 w524 w539 w553 w563 w574 w581]
                        tunnel: [w518 w534 w550 w559 w569 w577 w581] -> w505
                        tunnel: [w517 w535 w548 w560 w570 w572 "Cannot perform operation.\n" ("read buffer")] -> w504
                        tunnel: w509 -> [_ w528 w541 _ _ _ _]
                        frame "Serial Number" {
                          n152 = property on="Index" class="Ring (strict)"(error in=w513, "DisabledEnum"=T11."Disabled and Grayed Out" ("Disabled")) -> (error out=w512:errorcluster)  [unwired: 1 in, 1 out]
                          n153 = Concatenate Strings("SN" ("string"), "\r\n" ("write buffer")) -> (w516:string)
                          n154 = call "Serial.vi"("error in (no error)"=w512, "Clear Log"=FALSE, "write buffer"=w516, "VISA resource name"=w515) -> ("error out"=w518:errorcluster, "read buffer"=w517:string)  [unwired: 6 in]
                        }
                        frame "Temperature" {
                          n155 = Number To Decimal String(number=w528) -> (decimal integer string=w527:string)  [unwired: 1 in]
                          n156 = property on="Index" class="Ring (strict)"(error in=w524, "DisabledEnum"=T11."Enabled" ("Disabled"), "Visible"=TRUE) -> (error out=w523:errorcluster)  [unwired: 1 in, 1 out]
                          n157 = Concatenate Strings("TA" ("string"), "[", w527, "]", "\r\n" ("write buffer")) -> (w529:string)
                          n158 = call "Serial.vi"("error in (no error)"=w523, "Clear Log"=FALSE, "write buffer"=w529, "VISA resource name"=w533) -> ("error out"=w534:errorcluster, "read buffer"=w535:string)  [unwired: 6 in]
                        }
                        frame "Unit Adress" {
                          n159 = Number To Decimal String(number=w541) -> (decimal integer string=w547:string)  [unwired: 1 in]
                          n160 = property on="Index" class="Ring (strict)"(error in=w539, "DisabledEnum"=T11."Enabled" ("Disabled"), "Visible"=TRUE) -> (error out=w538:errorcluster)  [unwired: 1 in, 1 out]
                          n161 = Concatenate Strings("UA" ("string"), "[", w547, "]", "\r\n" ("write buffer")) -> (w542:string)
                          n162 = call "Serial.vi"("error in (no error)"=w538, "Clear Log"=FALSE, "write buffer"=w542, "VISA resource name"=w549) -> ("error out"=w550:errorcluster, "read buffer"=w548:string)  [unwired: 6 in]
                        }
                        frame "Calibration" {
                          n163 = property on="Index" class="Ring (strict)"(error in=w553, "DisabledEnum"=T11."Disabled and Grayed Out" ("Disabled")) -> (error out=w552:errorcluster)  [unwired: 1 in, 1 out]
                          n164 = Concatenate Strings("CC" ("string"), "\r\n" ("write buffer")) -> (w556:string)
                          n165 = call "Serial.vi"("error in (no error)"=w552, "Clear Log"=FALSE, "write buffer"=w556, "VISA resource name"=w558) -> ("error out"=w559:errorcluster, "read buffer"=w560:string)  [unwired: 6 in]
                        }
                        frame "Velocity" {
                          n166 = property on="Index" class="Ring (strict)"(error in=w563, "DisabledEnum"=T11."Disabled and Grayed Out" ("Disabled")) -> (error out=w562:errorcluster)  [unwired: 1 in, 1 out]
                          n167 = Concatenate Strings("VC" ("string"), "\r\n" ("write buffer")) -> (w566:string)
                          n168 = call "Serial.vi"("error in (no error)"=w562, "Clear Log"=FALSE, "write buffer"=w566, "VISA resource name"=w565) -> ("error out"=w569:errorcluster, "read buffer"=w570:string)  [unwired: 6 in]
                        }
                        frame "Version" {
                          n169 = Concatenate Strings("VR" ("string"), "\r\n" ("write buffer")) -> (w578:string)
                          n170 = property on="Index" class="Ring (strict)"(error in=w574, "DisabledEnum"=T11."Disabled and Grayed Out" ("Disabled")) -> (error out=w573:errorcluster)  [unwired: 1 in, 1 out]
                          n171 = call "Serial.vi"("error in (no error)"=w573, "Clear Log"=FALSE, "write buffer"=w578, "VISA resource name"=w576) -> ("error out"=w577:errorcluster, "read buffer"=w572:string)  [unwired: 6 in]
                        }
                        frame Default {
                        }
                      }
                      n172 = property on="Serial Send" class="Bool (strict)"(error in=w505, "Value"=FALSE ("Serial Send")) -> ()  [unwired: 1 in, 2 out]
                      n173 = property on="read buffer" class="Str"() -> ("Value"=w502:string)  [unwired: 2 in, 2 out]
                      n174 = Concatenate Strings(w502, w504) -> (w503:string)
                    }
                  }
                }
                frame "Set" {
                  n175 = To Unsigned Long Integer(number=w601) -> (unsigned 32bit integer=w597:u32)
                  n176 = Number To Decimal String(number=w596) -> (decimal integer string=w595:string)  [unwired: 1 in]
                  n177 = Number To Decimal String(number=w599) -> (decimal integer string=w598:string)  [unwired: 1 in]
                  n178 = case shown="Default" w592 {
                    tunnel: w591 -> [w676 w680 w684 w688 w692 w696 w698 w700]
                    tunnel: [FALSE TRUE TRUE FALSE FALSE FALSE w697 w699] -> w589
                    tunnel: [TRUE TRUE TRUE FALSE TRUE FALSE w697 w699] -> w588
                    tunnel: [FALSE FALSE FALSE TRUE FALSE FALSE w697 w699] -> w587
                    tunnel: [w676 w680 w684 w688 w692 w696 w698 w700] -> w585
                    frame "Serial Number" {
                    }
                    frame "Temperature" {
                    }
                    frame "Unit Adress" {
                    }
                    frame "Calibration" {
                    }
                    frame "Velocity" {
                    }
                    frame "Version" {
                    }
                    frame "Enable Conf. EP=1" {
                      w697 = FALSE
                    }
                    frame Default {
                      w699 = FALSE
                    }
                  }
                  n179 = Number To Decimal String(number=w597) -> (decimal integer string=w600:string)  [unwired: 1 in]
                  n180 = property on="Index" class="Ring (strict)"(error in=w585, "Visible"=w589) -> (error out=w590:errorcluster)  [unwired: 1 in, 1 out]
                  n181 = property on="Value" class="DigNum (strict)"(error in=w590, "Visible"=w588) -> (error out=w586:errorcluster)  [unwired: 1 in, 1 out]
                  n182 = property on="Value 1/2" class="Enum (strict)"(error in=w586, "Visible"=w587) -> (error out=w584:errorcluster)  [unwired: 1 in, 1 out]
                  n183 = case shown="True" w583 {
                    tunnel: w602 -> [_ w616]
                    tunnel: w600 -> [_ w615]
                    tunnel: w598 -> [_ w614]
                    tunnel: w597 -> [_ w613]
                    tunnel: w595 -> [_ w612]
                    tunnel: [w603 w611] -> w594
                    tunnel: [w604 w610] -> w593
                    tunnel: w592 -> [_ w608]
                    tunnel: w584 -> [w603 w607]
                    frame False {
                      n184 = property on="read buffer" class="Str"() -> ("Value"=w604:string)  [unwired: 2 in, 2 out]
                    }
                    frame True {
                      n185 = flat-sequence {
                        tunnel: [w620] -> w618
                        tunnel: w607 -> [w620]
                        frame #0 {
                          n186 = Wait (ms)(milliseconds to wait=u32 50) -> ()  [unwired: 1 out]
                        }
                      }
                      n187 = case shown="\"Velocity\"" w608 {
                        tunnel: [w623 w629 w638 w646 w664 "EP=1\r\n" ("write buffer") "Cannot perform operation.\n" ("read buffer")] -> w609
                        tunnel: w618 -> [w622 w628 w637 w651 w655 w667 w669]
                        tunnel: [w622 w628 w637 w651 w652 w667 w669] -> w617
                        tunnel: w615 -> [w624 w630 w643 _ _ _ _]
                        tunnel: w614 -> [_ _ _ w647 _ _ _]
                        tunnel: w613 -> [_ _ _ _ w656 _ _]
                        tunnel: w612 -> [_ w631 w641 _ _ _ _]
                        frame "Serial Number" {
                          n188 = Concatenate Strings("SN" ("write buffer"), "=" ("string"), w624, "\r\n" ("write buffer")) -> (w623:string)
                        }
                        frame "Temperature" {
                          n189 = Concatenate Strings("TA" ("string"), "[", w631, "]", "=" ("string"), w630, "\r\n" ("write buffer")) -> (w629:string)
                        }
                        frame "Unit Adress" {
                          n190 = Concatenate Strings("UA" ("string"), "[", w641, "]", "=" ("string"), w643, "\r\n" ("write buffer")) -> (w638:string)
                        }
                        frame "Calibration" {
                          n191 = Concatenate Strings("CC" ("string"), "=" ("string"), w647, "\r\n" ("write buffer")) -> (w646:string)
                        }
                        frame "Velocity" {
                          n192 = In Range and Coerce(upper limit=u16 18001, x=w656, lower limit=u16 0) -> (coerced(x)=w662:u32, In Range?=w660:bool)
                          n193 = Not(x=w660) -> (.not. x?=w661:bool)
                          n194 = Select(t=w662, s=w660, f=u16 0) -> (s? t:f=w654:u32)
                          n195 = Number To Decimal String(number=w654) -> (decimal integer string=w653:string)  [unwired: 1 in]
                          n196 = Concatenate Strings("VC" ("write buffer"), "=" ("string"), w653, "\r\n" ("write buffer")) -> (w664:string)
                          n197 = call "Display Message to User2"("error in (no error)"=w655, "Enable"=w661) -> ("error out"=w652:errorcluster)  [unwired: 8 in, 1 out]
                        }
                        frame "Enable Conf. EP=1" {
                        }
                        frame Default {
                        }
                      }
                      n198 = property on="read buffer" class="Str"() -> ("Value"=w605:string)  [unwired: 2 in, 2 out]
                      n199 = VISA Write(VISA resource name=w616, write buffer=w609, error in (no error)=w617) -> (error out=w619:errorcluster)  [unwired: 2 out]
                      n200 = Concatenate Strings(w605, w609) -> (w610:string)
                      n201 = property on="Serial Send" class="Bool (strict)"("Value"=FALSE ("Serial Send")) -> ()  [unwired: 2 in, 2 out]
                      n202 = flat-sequence {
                        tunnel: w619 -> [w671]
                        tunnel: [w671] -> w611
                        frame #0 {
                          n203 = Wait (ms)(milliseconds to wait=u32 50) -> ()  [unwired: 1 out]
                        }
                      }
                    }
                  }
                }
              }
              "read buffer" <- w457
              n204 = Add(x=u32 5, y=w450) -> (x+y=w449:u32)
              n205 = property on="read buffer" class="Str"(error in=w452, "Text.Scroll Position"=w449) -> (error out=w451:errorcluster)  [unwired: 1 in, 1 out]
            }
            event "Set Param.": Value Change {
              n206 = event-data() -> ()  [unwired: 1 in, 6 out]
              n207 = property on="Serial Status" class="Bool (strict)"(error in=w705) -> (error out=w704:errorcluster, "Value"=w709:bool)  [unwired: 1 in, 1 out]
              n208 = case shown="True" w709 {
                tunnel: w704 -> [w721 w734]
                tunnel: [w720 w730] -> w707
                frame False {
                  n209 = call "Display Message to User4"("error in (no error)"=w721) -> ("error out"=w720:errorcluster)  [unwired: 9 in, 1 out]
                }
                frame True {
                  w723 = FALSE ("Visible")
                  n210 = property on="Speed control" class="Bool (strict)"(error in=w734, "Visible"=FALSE) -> (error out=w733:errorcluster)  [unwired: 1 in, 1 out]
                  n211 = case shown="47" "Param to Set" {
                    tunnel: [w787 w791 w795] -> w749
                    tunnel: w733 -> [w786 w790 w794]
                    tunnel: [w786 w790 w794] -> w737
                    frame 95, Default {
                      n212 = call <vilib>:"Application Directory.vi"() -> ("Application Directory"=w789:path)
                      n213 = Build Path(base path=w789, name or relative path="data\\Marvin_EBAY_params_RRPAR000017_95_v0.2.txt") -> (appended path=w787:path)
                    }
                    frame 63 {
                      n214 = call <vilib>:"Application Directory.vi"() -> ("Application Directory"=w793:path)
                      n215 = Build Path(base path=w793, name or relative path="data\\Marvin_AHU_params_RRPAR000016_63_v0.2.txt") -> (appended path=w791:path)
                    }
                    frame 47 {
                      n216 = call <vilib>:"Application Directory.vi"() -> ("Application Directory"=w797:path)
                      n217 = Build Path(base path=w797, name or relative path="data\\Marvin_AHU_params_RRPAR000015_47_v0.2.txt") -> (appended path=w795:path)
                    }
                  }
                  n218 = property on="read buffer" class="Str"(error in=w737, "Visible"=TRUE) -> (error out=w725:errorcluster)  [unwired: 1 in, 1 out]
                  n219 = property on="CAN Data" class="Arr (strict)"(error in=w725, "Visible"=w723) -> (error out=w724:errorcluster)  [unwired: 1 in, 1 out]
                  n220 = property on="PlayPause Data Array" class="Bool (strict)"("Visible"=w723) -> ()  [unwired: 2 in, 2 out]
                  n221 = property on="Clear Data Array" class="Bool (strict)"("Visible"=w723) -> ()  [unwired: 2 in, 2 out]
                  n222 = property on="Horizontal Progress Bar" class="Slide (strict)"(error in=w724, "Visible"=TRUE, "Value"=u8 0 ("Horizontal Progress Bar")) -> (error out=w732:errorcluster)  [unwired: 1 in, 1 out]
                  n223 = call <vilib>:"Read Characters From File.vi"("file path (dialog if empty)"=w749) -> ("character string"=w750:string)  [unwired: 5 in, 3 out]
                  n224 = while {
                    shift-right: [w778] -> _
                    shift-left: w750 -> [w779]
                    shift-right: [w774] -> w735
                    shift-left: string[] [] -> [w775]
                    tunnel: w732 -> [w767]
                    tunnel: [w767] -> w747
                    stop <- w780 stop-if-true
                    n225 = Match Pattern(string=w779, regular expression="\r\n") -> (before substring=w776:string, after substring=w778:string, offset past match=w777:i32)  [unwired: 1 in, 1 out]
                    n226 = call <vilib>:"Trim Whitespace.vi"("string"=w776) -> ("trimmed string"=w773:string)  [unwired: 1 in]
                    n227 = Equal?(x=w777, y=-1) -> (x = y?=w780:bool)
                    n228 = To Upper Case(1:w773) -> (0:w771:string)
                    n229 = String Length(string=w771) -> (length=w770:i32)
                    n230 = Greater?(x=w770, y=3) -> (0:w768:bool)
                    n231 = case shown="True" w768 {
                      tunnel: w775 -> [w782 w785]
                      tunnel: [w782 w784] -> w774
                      tunnel: w771 -> [_ w783]
                      frame False {
                      }
                      frame True {
                        n232 = Build Array (concatenate)(w785, w783) -> (w784:string[])
                      }
                    }
                  }
                  n233 = property on="VISA resource name" class="VISAName"(error in=w747) -> (error out=w740:errorcluster, "Value"=w729:refnum<visa-resource-name>)  [unwired: 1 in, 1 out]
                  n234 = Build Array (concatenate)(w735, string[] ["MT", "VR", "SN"] ("array")) -> (w744:string[])
                  n235 = Array Size(array=w744) -> (size(s)=w736:i32)
                  n236 = Bundle By Name(cluster=T12 {"Minimum"=0.0, "Maximum"=0.0, "Increment"=0.0} ("Data Entry Limits"), "Minimum"=0.0, "Maximum"=w736) -> (w742:T12)
                  n237 = property on="Horizontal Progress Bar" class="Slide (strict)"(error in=w740, "Data Range"=w742) -> (error out=w728:errorcluster)  [unwired: 1 in, 1 out]
                  n238 = property on="read buffer" class="Str"(error in=w728) -> (error out=w727:errorcluster, "Text.Scroll Position"=w726:u32)  [unwired: 1 in, 1 out]
                  n239 = for {
                    tunnel: w744 -> [w758] mode=indexing
                    tunnel: w729 -> [w764]
                    tunnel: w727 -> [w763]
                    tunnel: [w755] -> w731
                    tunnel: w726 -> [w754]
                    i -> [w753]
                    n240 = Concatenate Strings(w758, "\r\n" ("string")) -> (w756:string)
                    n241 = VISA Write(VISA resource name=w764, write buffer=w756, error in (no error)=w763) -> (error out=w762:errorcluster)  [unwired: 2 out]
                    n242 = flat-sequence {
                      tunnel: w762 -> [w765]
                      tunnel: [w765] -> w755
                      frame #0 {
                        n243 = Wait (ms)(milliseconds to wait=u32 50) -> ()  [unwired: 1 out]
                      }
                    }
                    n244 = Add(x=w754, y=w753) -> (x+y=w752:u32)
                    n245 = feedback #1("") -> (w760:string)
                    n246 = Concatenate Strings(w760, w756) -> (w761:string)
                    n247 = feedback-in #1(w761) -> ()
                    n248 = property on="read buffer" class="Str"("Value"=w761, "Text.Scroll Position"=w752) -> ()  [unwired: 2 in, 2 out]
                    "Horizontal Progress Bar" <- w753
                  }
                  n249 = VISA Flush I/O Buffer(VISA resource name=w729, error in (no error)=w731) -> (error out=w730:errorcluster)  [unwired: 1 in, 1 out]
                }
              }
              n250 = property on="Serial Monitor" class="Bool (strict)"(error in=w707) -> (error out=w706:errorcluster, "Value"=w708:bool)  [unwired: 1 in, 1 out]
              n251 = case shown="False" w708 {
                tunnel: w706 -> [w718 w719]
                tunnel: [w715 w719] -> w702
                frame False {
                  w714 = TRUE ("Visible")
                  n252 = property on="PlayPause Data Array" class="Bool (strict)"("Visible"=w714) -> ()  [unwired: 2 in, 2 out]
                  n253 = property on="read buffer" class="Str"(error in=w718, "Visible"=FALSE) -> (error out=w716:errorcluster)  [unwired: 1 in, 1 out]
                  n254 = property on="Clear Data Array" class="Bool (strict)"("Visible"=w714) -> ()  [unwired: 2 in, 2 out]
                  n255 = property on="CAN Data" class="Arr (strict)"(error in=w716, "Visible"=w714) -> (error out=w715:errorcluster)  [unwired: 1 in, 1 out]
                }
                frame True {
                }
              }
              n256 = call "Display Message to User5"("error in (no error)"=w702) -> ("error out"=w701:errorcluster)  [unwired: 9 in, 1 out]
            }
            event "Help Button": Value Change {
              n257 = event-data() -> ()  [unwired: 1 in, 6 out]
              n258 = control-ref of="This VI"() -> (w806:refnum<vi>)
              n259 = property class="VI"(reference=w806, error in=w804, "FP:Transparency"=u8 25 ("Front Panel Window:Transparency")) -> (reference out=w800:refnum<vi>, error out=w803:errorcluster)
              n260 = vi-ref "Help.vi"() -> (w810:refnum<vi>)
              n261 = invoke class="VI" method="FP.Open"(reference=w810, error in=w803, "Activate"=TRUE ("Activate?"), "State"=T13."Standard") -> (error out=w809:errorcluster)  [unwired: 1 in, 4 out]
              n262 = call "Help.vi"("error in"=w809, "TesterSWVersion"="1.7") -> ("error out"=w802:errorcluster)  [unwired: 6 in]
              n263 = property class="VI"(reference=w800, error in=w802, "FP:Transparency"=u8 0 ("Front Panel Window:Transparency")) -> (error out=w801:errorcluster)  [unwired: 1 out]
            }
            event "Can Send": Value Change {
              w845 = u8 0 items=["STATUS"=128, "EXTENDED"=2, "RTR"=1, "DATA MSG"=0] ("MSGTYPE")
              w850 = u8 1 items=["Standart flag", "Extern flag"] ("Format")
              w849 = u8 0 items=["Data flag", "Remote flag"] ("Type")
              # "Send"
              n264 = event-data() -> ()  [unwired: 1 in, 6 out]
              n265 = In Range and Coerce(upper limit=u16 18001, x="Motor Speed RPM", lower limit=u16 0) -> (coerced(x)=w832:u16, In Range?=w830:bool)
              n266 = In Range and Coerce(upper limit=u16 100, x="Motor Phase Current", lower limit=u16 40) -> (coerced(x)=w821:u16, In Range?=w823:bool)
              n267 = Not(x=w830) -> (.not. x?=w831:bool)
              n268 = Not(x=w823) -> (.not. x?=w822:bool)
              n269 = call "Display Message to User"("Enable"=w831) -> ()  [unwired: 9 in, 2 out]
              n270 = Select(t=w832, s=w830, f=u16 0) -> (s? t:f=w834:u16)
              n271 = call "Display Message to User6"("Enable"=w822) -> ()  [unwired: 9 in, 2 out]
              n272 = Select(t=w821, s=w823, f=u16 0) -> (s? t:f=w816:u16)
              n273 = property on="UUT" class="DigNum (strict)"() -> ("Value"=w828:u8)  [unwired: 2 in, 2 out]
              n274 = Split Number(x=w834) -> (hi(x)=w837:u8, lo(x)=w838:u8)
              n275 = case shown="79" w828 {
                tunnel: [u32 417357607 u32 417353511 u32 417349415 u32 417345319] -> w829
                frame 95, Default {
                }
                frame 79 {
                }
                frame 63 {
                }
                frame 47 {
                }
              }
              n276 = case shown="79" w828 {
                tunnel: [w869 w878 w891 w905] -> w843
                tunnel: w838 -> [w868 w877 w890 w904]
                tunnel: w837 -> [w867 w876 w889 w903]
                tunnel: "Motor Speed RPM" -> [w864 w873 _ _]
                tunnel: "Speed control" -> [_ _ w882 w896]
                tunnel: "Motor Over Temp" -> [_ _ w881 w895]
                tunnel: w816 -> [_ _ _ w892]
                frame 47, Default {
                  w866 = u8 0 ("element")
                  n277 = case shown="1, Default" w864 {
                    tunnel: [u8 1 ("element") u8 0 ("element")] -> w863
                    frame 1, Default {
                    }
                    frame 0 {
                    }
                  }
                  n278 = Build Array(u8 1 ("element"), w868, w867, w863, w866, w866, w866, w866) -> (w869:u8[])
                }
                frame 63 {
                  w874 = u8 0 ("element")
                  n279 = case shown="1, Default" w873 {
                    tunnel: [u8 1 ("element") u8 0 ("element")] -> w872
                    frame 1, Default {
                    }
                    frame 0 {
                    }
                  }
                  n280 = Build Array(u8 1 ("element"), w877, w876, w872, w874, w874, w874, w874) -> (w878:u8[])
                }
                frame 95 {
                  w887 = u8 0 ("element")
                  n281 = Boolean To (0,1)(Boolean=w882) -> (0, 1=w885:i16)
                  n282 = Boolean To (0,1)(Boolean=w881) -> (0, 1=w886:i16)
                  n283 = To Unsigned Byte Integer(number=w885) -> (unsigned 8bit integer=w884:u8)
                  n284 = To Unsigned Byte Integer(number=w886) -> (unsigned 8bit integer=w883:u8)
                  n285 = Build Array(u8 1 ("element"), w890, w889, w884, w883, w887, w887, w887) -> (w891:u8[])
                }
                frame 79 {
                  n286 = Split Number(x=w892) -> (hi(x)=w893:u8, lo(x)=w894:u8)
                  n287 = Boolean To (0,1)(Boolean=w896) -> (0, 1=w899:i16)
                  n288 = Boolean To (0,1)(Boolean=w895) -> (0, 1=w900:i16)
                  n289 = To Unsigned Byte Integer(number=w899) -> (unsigned 8bit integer=w898:u8)
                  n290 = To Unsigned Byte Integer(number=w900) -> (unsigned 8bit integer=w897:u8)
                  n291 = Build Array(u8 1 ("element"), w904, w903, w898, w897, w894, w893, u8 0 ("element")) -> (w905:u8[])
                }
              }
              n292 = Array Size(array=w843) -> (size(s)=w848:i32)
              n293 = call "Array Data to Single Num in Hex.vi"("aDATA"=w843) -> ("Numeric"=→"Data Send":u64)  [unwired: 10 in]
              n294 = To Unsigned Byte Integer(number=w848) -> (unsigned 8bit integer=w846:u8)
              n295 = call "CANAnalData.vi"("ID"=w829, "Data"=w843, "Config"=w841) -> ()  [unwired: 4 in, 5 out]
              n296 = Bundle By Name(cluster=T10 {"ID"=0, "MSGTYPE"=0, "LEN"=0, "aDATA"=[]} ("MsgTX 2"), "ID"=w829, "MSGTYPE"=w845, "LEN"=w846, "aDATA"=w843) -> (w844:T10)
              n297 = Unbundle By Name(w844) -> ("ID"=w858:u32, "LEN"=w859:u8, "aDATA"=w860:u8[])  [unwired: 1 out]
              n298 = property class="Clust (strict)"(reference=w841) -> ("Value"=w857:T8)  [unwired: 1 in, 2 out]
              n299 = Bundle By Name(cluster=T14 {"ID"=0, "TimeStamp"=0, "TimeFlag"=0, "SendType"=0, "RemoteFlag"=0, "ExternFlag"=0, "DataLen"=0, "Data"=[], "Reserved"=[]} ("Send"), "ID"=w858, "RemoteFlag"=w849, "ExternFlag"=w850, "DataLen"=w859, "Data"=w860) -> (w855:T14)
              n300 = Unbundle By Name(w857) -> ("DevType"=w851:T2, "DevIndex"=w852:u32, "CanIndex"=w853:T3)
              n301 = Build Array(w855) -> (w854:T14[])
              n302 = call "VCI_Transmit.vi"("Buffer"=w854, "CANIndex"=w853, "DevIndex"=w852, "DevType"=w851) -> ()  [unwired: 1 in, 7 out]
            }
            event "Graph Button": Value Change {
              w910 = FALSE ("Visible")
              n303 = event-data() -> ()  [unwired: 1 in, 6 out]
              n304 = Not(x="Graph Button") -> (.not. x?=w911:bool)
              n305 = property on="PlayPause Data Array" class="Bool (strict)"("Visible"=w911) -> ()  [unwired: 2 in, 2 out]
              n306 = property on="CAN Data" class="Arr (strict)"(error in=w912, "Visible"=w911) -> (error out=w913:errorcluster)  [unwired: 1 in, 1 out]
              n307 = property on="Clear Data Array" class="Bool (strict)"("Visible"=w911) -> ()  [unwired: 2 in, 2 out]
              n308 = property on="Waveform Chart" class="WFChart (strict)"(error in=w913, "Visible"="Graph Button") -> (error out=w915:errorcluster)  [unwired: 1 in, 1 out]
              n309 = property on="Serial Monitor" class="Bool (strict)"(error in=w915) -> (error out=w929:errorcluster, "Value"=w930:bool)  [unwired: 1 in, 1 out]
              n310 = case shown="True" w930 {
                tunnel: w929 -> [w937 w942]
                tunnel: [w935 w939] -> w918
                frame False {
                  n311 = property on="read buffer" class="Str"(error in=w937, "Visible"=FALSE) -> (error out=w935:errorcluster)  [unwired: 1 in, 1 out]
                }
                frame True {
                  w938 = FALSE ("Visible")
                  n312 = property on="PlayPause Data Array" class="Bool (strict)"("Visible"=w938) -> ()  [unwired: 2 in, 2 out]
                  n313 = property on="read buffer" class="Str"(error in=w942, "Visible"=TRUE) -> (error out=w940:errorcluster)  [unwired: 1 in, 1 out]
                  n314 = property on="Clear Data Array" class="Bool (strict)"("Visible"=w938) -> ()  [unwired: 2 in, 2 out]
                  n315 = property on="CAN Data" class="Arr (strict)"(error in=w940, "Visible"=w938) -> (error out=w939:errorcluster)  [unwired: 1 in, 1 out]
                }
              }
              n316 = property on="Serial Monitor" class="Bool (strict)"(error in=w918, "Value"=FALSE ("Serial Monitor")) -> (error out=w916:errorcluster)  [unwired: 1 in, 1 out]
              n317 = property on="Index" class="Ring (strict)"(error in=w916, "Visible"=w910) -> (error out=w926:errorcluster)  [unwired: 1 in, 1 out]
              n318 = property on="Value 1/2" class="Enum (strict)"(error in=w926, "Visible"=w910) -> (error out=w925:errorcluster)  [unwired: 1 in, 1 out]
              n319 = property on="Value" class="DigNum (strict)"(error in=w925, "Visible"=w910) -> (error out=w924:errorcluster)  [unwired: 1 in, 1 out]
              n320 = property on="SetGet" class="Enum (strict)"(error in=w924, "Visible"=w910) -> (error out=w923:errorcluster)  [unwired: 1 in, 1 out]
              n321 = property on="Serial Send" class="Bool (strict)"(error in=w923, "Visible"=w910) -> (error out=w921:errorcluster)  [unwired: 1 in, 1 out]
              n322 = property on="Clear Monitor" class="Bool"(error in=w921, "Visible"=w910) -> (error out=w920:errorcluster)  [unwired: 1 in, 1 out]
              n323 = property on="Function" class="Enum (strict)"(error in=w920, "Visible"=w910) -> (error out=w922:errorcluster)  [unwired: 1 in, 1 out]
              n324 = property on="Index" class="Ring (strict)"(error in=w922, "Visible"=w910) -> (error out=w927:errorcluster)  [unwired: 1 in, 1 out]
              n325 = property on="read buffer" class="Str"(error in=w927, "Visible"=w910) -> (error out=w919:errorcluster)  [unwired: 1 in, 1 out]
            }
            event "Serial Com": Value Change {
              n326 = event-data() -> ()  [unwired: 1 in, 6 out]
              n327 = property on="Serial Com" class="Bool"(error in=w947, "Visible"=FALSE) -> (error out=w946:errorcluster)  [unwired: 1 in, 1 out]
              n328 = property on="VISA resource name" class="VISAName"(error in=w946, "Visible"=TRUE) -> (error out=w944:errorcluster)  [unwired: 1 in, 1 out]
            }
            event "VISA resource name": Value Change {
              n329 = event-data() -> ()  [unwired: 1 in, 1 out]
              n330 = control-ref of="This VI"() -> (w953:refnum<vi>)
              n331 = call "Serial InitMarvin.vi"("error in (no error)"=w962, "VI reference (current VI)"=w953, "VISA Refnum in"="VISA resource name") -> ("error out"=w971:errorcluster, "Boolean"=w959:bool)  [unwired: 7 in]
              n332 = property on="Serial Status" class="Bool (strict)"(error in=w971, "Value"=w959) -> (error out=w965:errorcluster)  [unwired: 1 in, 1 out]
              n333 = property on="VISA resource name" class="VISAName"(error in=w965, "Visible"=FALSE) -> (error out=w964:errorcluster)  [unwired: 1 in, 1 out]
              n334 = property on="Serial Com" class="Bool"(error in=w964, "Visible"=TRUE) -> (error out=w957:errorcluster)  [unwired: 1 in, 1 out]
              n335 = call "Serial.vi"("error in (no error)"=w957, "Clear Log"=TRUE, "VISA resource name"="VISA resource name") -> ("error out"=w955:errorcluster)  [unwired: 7 in, 1 out]
              n336 = call <vilib>:"Clear Errors.vi"("error in (no error)"=w955) -> ("error out"=w961:errorcluster)  [unwired: 5 in, 1 out]
              n337 = case shown="True" w959 {
                tunnel: w961 -> [w972 w975]
                tunnel: [w972 w974] -> w960
                tunnel: "VISA resource name" -> [_ w973]
                frame False {
                }
                frame True {
                  n338 = VISA Flush I/O Buffer(VISA resource name=w973, error in (no error)=w975) -> (error out=w974:errorcluster)  [unwired: 1 in, 1 out]
                }
              }
            }
            event "Stop": Value Change {
              n339 = event-data() -> ()  [unwired: 1 in, 6 out]
              n340 = Flush Queue(queue=w981, error in (no error)=w980) -> (queue out=w979:refnum<queue>, error out=w978:errorcluster)  [unwired: 1 out]
              n341 = Release Queue(queue=w979, error in (no error)=w978) -> (error out=w977:errorcluster)  [unwired: 1 in, 2 out]
            }
            event "Refresh Button": Value Change {
              n342 = event-data() -> ()  [unwired: 1 in, 6 out]
              n343 = Release Queue(queue=w987, error in (no error)=w988) -> (error out=w986:errorcluster)  [unwired: 1 in, 2 out]
            }
          }
          n344 = Unbundle By Name(w268) -> ("status"=w274:bool)
          n345 = Or(x=w274, y=w266) -> (x .or. y?=w273:bool)
        }
        n346 = while {
          shift-right: [w120] -> _
          shift-left: w98 -> [w122]
          shift-right: [w118] -> _
          shift-left: _ -> [w119]
          shift-right: [w114] -> _
          shift-left: w97 -> [w114]
          shift-right: [w113] -> w93
          shift-left: w94 -> [w112]
          shift-right: [w105] -> _
          shift-left: cluster{"Frame Data":u64, "Frame ID":u32}[] [] ("Array 3") -> [w107]
          stop <- w121 stop-if-true
          n347 = Dequeue Element(queue=w122, error in (no error)=w114) -> (queue out=w120:refnum<queue>, element=w115:T9, error out=w121:errorcluster)  [unwired: 1 in, 1 out]
          n348 = for {
            tunnel: [w252] -> w117 mode=indexing
            tunnel: w115 -> [w254] mode=indexing
            tunnel: [w253] -> w116 mode=indexing
            tunnel: [w251] -> w111 mode=indexing
            tunnel: [w250] -> w110 mode=indexing
            shift-right: [w250] -> _
            shift-left: _ -> [w249]
            n349 = Unbundle By Name(w254) -> ("ID"=w251:u32, "aDATA"=w253:u8[])
            n350 = call "Array Data to Single Num in Hex.vi"("aDATA"=w253) -> ("Numeric"=w252:u64)  [unwired: 10 in]
            n351 = case shown="Default" w251 {
              tunnel: w252 -> [_ w259]
              tunnel: w251 -> [_ w258]
              tunnel: [w255 w257] -> w250
              tunnel: w249 -> [w255 _]
              frame 0 {
              }
              frame Default {
                n352 = Bundle By Name(cluster=cluster{"Frame Data":u64, "Frame ID":u32} {"Frame Data"=0, "Frame ID"=0} ("Cluster"), "Frame ID"=w258, "Frame Data"=w259) -> (w257:cluster{"Frame Data":u64, "Frame ID":u32})
              }
            }
          }
          n353 = case shown="True" "PlayPause Data Array" {
            tunnel: w110 -> [w125 _]
            tunnel: w107 -> [w124 w126]
            tunnel: [w123 w126] -> w106
            frame False {
              n354 = Build Array (concatenate)(w125, w124) -> (w123:cluster{"Frame Data":u64, "Frame ID":u32}[])
            }
            frame True {
            }
          }
          n355 = Build Array (concatenate)(w117, w119) -> (w118:u64[][])
          "Array" <- w118
          n356 = Select(t=cluster{"Frame Data":u64, "Frame ID":u32}[] [], s="Clear Data Array", f=w106) -> (s? t:f=w105:cluster{"Frame Data":u64, "Frame ID":u32}[])
          "CAN Data" <- w105
          n357 = for {
            tunnel: w116 -> [w130] mode=indexing
            tunnel: [w129] -> w113
            tunnel: w112 -> [w128]
            tunnel: w111 -> [w127] mode=indexing
            n358 = case shown="417408831, 417408847, 417408863" w127 {
              tunnel: w130 -> [_ w160 w198 w248]
              tunnel: [w131 w137 w189 w239] -> w129
              tunnel: w128 -> [w131 w136 w189 w239]
              frame Default {
              }
              frame 417408831, 417408847, 417408863 {
                # "Frame ID\n0x18E1273F"
                n359 = Index Array(array=w160, index #1=0 ("index"), index #2=1 ("index"), index #3=2 ("index"), index #4=3 ("index"), index #5=4 ("index"), index #6=5 ("index"), index #7=6 ("index"), index #8=7 ("index")) -> (element #1=w144:u8, element #2=w146:u8, element #3=w147:u8, element #4=w151:u8, element #5=w154:u8, element #6=w158:u8, element #7=w159:u8, element #8=w157:u8)
                n360 = Join Numbers(hi=w159, lo=w158) -> ((hi.lo)=w178:u16)
                n361 = Join Numbers(hi=w147, lo=w146) -> ((hi.lo)=w148:u16)
                n362 = Number To Hexadecimal String(2:w178) -> (0:w177:string)  [unwired: 1 in]
                n363 = Number To Hexadecimal String(2:w157) -> (0:w171:string)  [unwired: 1 in]
                n364 = Number To Hexadecimal String(2:w144) -> (0:w145:string)  [unwired: 1 in]
                n365 = Number To Hexadecimal String(2:w148) -> (0:w149:string)  [unwired: 1 in]
                n366 = Number To Hexadecimal String(2:w151) -> (0:w152:string)  [unwired: 1 in]
                n367 = Number To Hexadecimal String(2:w154) -> (0:w155:string)  [unwired: 1 in]
                n368 = Hexadecimal String To Number(string=w145) -> (number=w142:u32)  [unwired: 2 in, 1 out]
                n369 = Hexadecimal String To Number(string=w149) -> (number=w150:u32)  [unwired: 2 in, 1 out]
                n370 = Hexadecimal String To Number(string=w152) -> (number=w153:u32)  [unwired: 2 in, 1 out]
                n371 = Hexadecimal String To Number(string=w155) -> (number=w156:u32)  [unwired: 2 in, 1 out]
                n372 = Hexadecimal String To Number(string=w171) -> (number=w170:u32)  [unwired: 2 in, 1 out]
                n373 = Hexadecimal String To Number(string=w177) -> (number=w176:u32)  [unwired: 2 in, 1 out]
                n374 = To Unsigned Word Integer(number=w142) -> (unsigned 16bit integer=→"ECS State":u16)
                n375 = To Double Precision Float(number=w150) -> (double precision float=w134:dbl)
                "Motor Speed RPM" <- w134
                n376 = To Double Precision Float(number=w176) -> (double precision float=w173:dbl)
                n377 = To Double Precision Float(number=w170) -> (double precision float=→"DC Current":dbl)
                n378 = To Double Precision Float(number=w153) -> (double precision float=w141:dbl)
                n379 = To Double Precision Float(number=w156) -> (double precision float=w139:dbl)
                n380 = To Double Precision Float(number=u32 10 ("y")) -> (double precision float=w174:dbl)
                n381 = Subtract(x=w139, y=50.0 ("x")) -> (x-y=→"Power transistor Heat sink Temp.":dbl)
                n382 = Subtract(x=w141, y=50.0 ("x")) -> (x-y=→"Motor Stator Temp.":dbl)
                n383 = Divide(x=w173, y=w174) -> (x/y=→"DC Voltage":dbl)
                n384 = case shown="True" TRUE {
                  tunnel: w136 -> [w179 w182]
                  tunnel: [w179 w181] -> w137
                  tunnel: w134 -> [_ w180]
                  frame False {
                  }
                  frame True {
                    n385 = disable-structure shown="Disabled" {
                      disable-tunnel: w180 -> [w186 _]
                      frame Disabled {
                        n386 = call <vilib>:"Application Directory.vi"() -> ("Application Directory"=w184:path)
                        n387 = Build Path(base path=w184, name or relative path="RPM Log.lvm") -> (appended path=w185:path)
                        n388 = call "Write To Measurement File"("Signals"=w186, "Filename"=w185) -> ()  [unwired: 15 in, 3 out]
                      }
                      frame Enabled {
                      }
                    }
                    n389 = Build Array (concatenate)(w180, w182) -> (w181:dbl[])
                    "Waveform Chart" <- w181
                  }
                }
              }
              frame 417539903, 417539919, 417539935 {
                # "Framde ID\n0x18E3273F"
                n390 = property on="UUT" class="DigNum (strict)"() -> ("Value"=w188:u8)  [unwired: 2 in, 2 out]
                n391 = Index Array(array=w198, index #1=0 ("index"), index #2=1 ("index")) -> (element #1=w196:u8, element #2=w191:u8)
                n392 = case shown="Default" w188 {
                  tunnel: [0 1 2] -> w187
                  frame Default {
                  }
                  frame 95 {
                  }
                  frame 79 {
                  }
                }
                n393 = Number To Boolean Array(number=w196) -> (Boolean array=w195:bool[])
                n394 = Number To Boolean Array(number=w191) -> (Boolean array=w193:bool[])
                n395 = Boolean To (0,1)(Boolean=w193) -> (0, 1=w190:i16[])
                n396 = Boolean To (0,1)(Boolean=w195) -> (0, 1=w194:i16[])
                n397 = case shown="79, 95" w188 {
                  tunnel: w190 -> [_ w203]
                  tunnel: w187 -> [_ w202]
                  frame 0, Default {
                  }
                  frame 79, 95 {
                    n398 = for {
                      tunnel: w203 -> [w208] mode=indexing
                      tunnel: w202 -> [w204]
                      i -> [w205]
                      stop <- w206 stop-if-true
                      n399 = Not Equal To 0?(x=w208) -> (x != 0?=w207:bool)
                      n400 = case shown="2" w205 {
                        tunnel: w207 -> [w209 w210 w211]
                        frame 0, Default {
                          "Ambient Sensor temp" <- w209
                        }
                        frame 1 {
                          "Ambient Over temp" <- w210
                        }
                        frame 2 {
                          "Hall Sensor Fault" <- w211
                        }
                      }
                      n401 = Equal?(x=w205, y=w204) -> (x = y?=w206:bool)
                    }
                  }
                }
                n402 = for {
                  tunnel: w194 -> [w213] mode=indexing
                  i -> [w214]
                  n403 = Not Equal To 0?(x=w213) -> (x != 0?=w212:bool)
                  n404 = case shown="0, Default" w214 {
                    tunnel: w212 -> [w215 w216 w217 w218 w219 w220 w221 w222]
                    frame 0, Default {
                      "Drive Sensor temp Failure" <- w215
                    }
                    frame 1 {
                      "Drive Over temperature" <- w216
                    }
                    frame 2 {
                      "Motor Sensor temp Fauilre" <- w217
                    }
                    frame 3 {
                      "Motor Over temperature" <- w218
                    }
                    frame 4 {
                      "Derated drive temp" <- w219
                    }
                    frame 5 {
                      "Under voltage/Over voltage" <- w220
                    }
                    frame 6 {
                      "Commutation err" <- w221
                    }
                    frame 7 {
                      "Speed error" <- w222
                    }
                  }
                }
              }
              frame 417474367, 417474383, 417474399 {
                w230 = "."
                # "Frame ID\n0x18E2273F"
                n405 = Index Array(array=w248, index #1=0 ("index")) -> (element #1=w246:u8, element #2=w244:u8, element #3=w224:u8, element #4=w225:u8, element #5=w226:u8, element #6=w227:u8)  [unwired: 5 in]
                n406 = Split Number(x=w226) -> (hi(x)=w238:u8, lo(x)=w237:u8)
                n407 = Split Number(x=w227) -> (hi(x)=w236:u8, lo(x)=w235:u8)
                n408 = Join Numbers(hi=w225, lo=w224) -> ((hi.lo)=→"Motor Phase Current":u16)
                n409 = Number To Decimal String(number=w238) -> (decimal integer string=w234:string)  [unwired: 1 in]
                n410 = Number To Decimal String(number=w237) -> (decimal integer string=w233:string)  [unwired: 1 in]
                n411 = Number To Decimal String(number=w236) -> (decimal integer string=w232:string)  [unwired: 1 in]
                n412 = Number To Decimal String(number=w235) -> (decimal integer string=w231:string)  [unwired: 1 in]
                n413 = Concatenate Strings(w234, w230, w233, w230, w232, w230, w231) -> (→"Driver Version":string)
                n414 = Number To Hexadecimal String(2:w244) -> (0:w242:string)  [unwired: 1 in]
                n415 = Hexadecimal String To Number(string=w242) -> (number=w243:u32)  [unwired: 2 in, 1 out]
                n416 = To Double Precision Float(number=w243) -> (double precision float=w241:dbl)
                n417 = Subtract(x=w241, y=50.0) -> (x-y=→"Ambient Temperature":dbl)
                n418 = To Double Precision Float(number=w246) -> (double precision float=→"Motor Phase Current RMS":dbl)
              }
            }
          }
        }
      }
      frame "Stop" {
        n419 = Release Queue(queue=w996, error in (no error)=w998) -> (error out=w997:errorcluster)  [unwired: 1 in, 2 out]
        n420 = flat-sequence {
          tunnel: w995 -> [w999]
          tunnel: [TRUE ("Stop")] -> w994
          frame #0 {
            w1005 = u8[] [1, 0, 0, 0, 0, 0, 0, 0] ("Data 2")
            w1007 = u8 0 items=["STATUS"=128, "EXTENDED"=2, "RTR"=1, "DATA MSG"=0] ("MSGTYPE")
            w1012 = u8 1 items=["Standart flag", "Extern flag"] ("Format")
            w1011 = u8 0 items=["Data flag", "Remote flag"] ("Type")
            n421 = property on="Serial Status" class="Bool (strict)"() -> ("Value"=w1000:bool)  [unwired: 2 in, 2 out]
            n422 = property on="UUT" class="DigNum (strict)"() -> ("Value"=w1002:u8)  [unwired: 2 in, 2 out]
            n423 = case shown="True" w1000 {
              frame False {
              }
              frame True {
                n424 = property on="VISA resource name" class="VISAName"() -> ("Value"=w1023:refnum<visa-resource-name>)  [unwired: 2 in, 2 out]
                n425 = VISA Close(VISA resource name=w1023) -> ()  [unwired: 1 in, 1 out]
              }
            }
            n426 = case shown="95, Default" w1002 {
              tunnel: [u32 417357607 u32 417349415 u32 417345319] -> w1001
              frame 95, Default {
              }
              frame 63 {
              }
              frame 47 {
              }
            }
            n427 = property on="Graph Button" class="Bool (strict)"("Value"=FALSE ("Graph Button")) -> ()  [unwired: 2 in, 2 out]
            n428 = Array Size(array=w1005) -> (size(s)=w1010:i32)
            n429 = To Unsigned Byte Integer(number=w1010) -> (unsigned 8bit integer=w1008:u8)
            n430 = Bundle By Name(cluster=T10 {"ID"=0, "MSGTYPE"=0, "LEN"=0, "aDATA"=[]} ("MsgTX 2"), "ID"=w1001, "MSGTYPE"=w1007, "LEN"=w1008, "aDATA"=w1005) -> (w1006:T10)
            n431 = call "CANAnalData.vi"("ID"=w1001, "Data"=w1005, "Config"=w999) -> ()  [unwired: 4 in, 5 out]
            n432 = call "Array Data to Single Num in Hex.vi"("aDATA"=w1005) -> ("Numeric"=w1004:u64)  [unwired: 10 in]
            n433 = property on="Data Send" class="DigNum (strict)"("Value"=w1004) -> ()  [unwired: 2 in, 2 out]
            n434 = Unbundle By Name(w1006) -> ("ID"=w1020:u32, "LEN"=w1021:u8, "aDATA"=w1022:u8[])  [unwired: 1 out]
            n435 = property class="Clust (strict)"(reference=w999) -> ("Value"=w1019:T8)  [unwired: 1 in, 2 out]
            n436 = Bundle By Name(cluster=T14 {"ID"=0, "TimeStamp"=0, "TimeFlag"=0, "SendType"=0, "RemoteFlag"=0, "ExternFlag"=0, "DataLen"=0, "Data"=[], "Reserved"=[]} ("Send"), "ID"=w1020, "RemoteFlag"=w1011, "ExternFlag"=w1012, "DataLen"=w1021, "Data"=w1022) -> (w1017:T14)
            n437 = Unbundle By Name(w1019) -> ("DevType"=w1013:T2, "DevIndex"=w1014:u32, "CanIndex"=w1015:T3)
            n438 = Build Array(w1017) -> (w1016:T14[])
            n439 = call "VCI_Transmit.vi"("Buffer"=w1016, "CANIndex"=w1015, "DevIndex"=w1014, "DevType"=w1013) -> ()  [unwired: 1 in, 7 out]
          }
          frame #1 {
          }
        }
      }
    }
  }
  n440 = disable-structure shown="Disabled" {
    frame Disabled {
      n441 = control-ref of="Config_CANAT"() -> ()  [unwired: 1 out]
      n442 = control-ref of="UUT"() -> ()  [unwired: 1 out]
    }
    frame Enabled {
    }
  }
